vi "WPI_AnalogChannelGetSampleRate.vi"(8 "error in (no error)":errorcluster) -> (0 "error out":errorcluster, 1 "Scan List":u8[](array[numeric]), 2 "Samples Per Second":dbl)   [LabVIEW 2017]
doc: "Returns the sample rate. The effective sample rate for a channel is the sample rate divided by the number of active channels. Use the SetSampleRate VI to set the sample rate of a channel.\n\nThis software is licensed. Open the labview\\readme\\WPI Robotics Library Open Source License.txt file for more information."
uses:
  <vilib>/Rock Robotics/SystemInterfaces/System/FPGA_SystemGet.vi
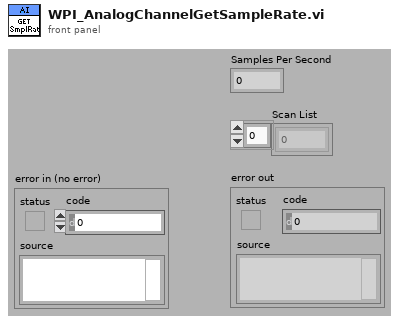
[diagram p1: front panel]
types:
  T1 = typedef "FPGA_AIDevRef.ctl" = cluster{"DevStatus":errorcluster}
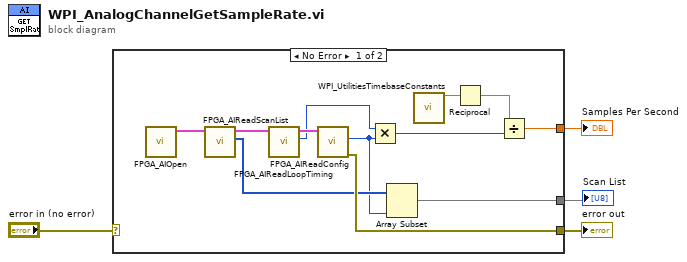
[diagram p0: block diagram]
diagram:
  n1 = case shown="No Error" "error in (no error)" {
    selector: "error in (no error)" -> [_ w17]
    tunnel: [w12 w17] -> w3
    tunnel: [w13 _] -> w2
    tunnel: [w8 _] -> w1
    frame No Error {
      n2 = call <vilib>:"FPGA_AIOpen.vi"() -> ("AI Reference out"=w11:T1)  [unwired: 3 in, 8 out]
      n3 = call <vilib>:"FPGA_AIReadScanList.vi"("AI Reference"=w11) -> ("Scan List"=w9:u8[], "AI Reference"=w10:T1)  [unwired: 1 in, 8 out]
      n4 = call <vilib>:"FPGA_AIReadLoopTiming.vi"("AI Reference"=w10) -> ("LoopTiming"=w15:u32, "AI Reference"=w16:T1)  [unwired: 1 in, 8 out]
      n5 = call <vilib>:"FPGA_AIReadConfig.vi"("AI Reference"=w16) -> ("error out"=w12:errorcluster, "Scan Size"=w7:u8)  [unwired: 1 in, 8 out]
      n6 = Multiply(x=w15, y=w7) -> (x*y=w14:u32)
      n7 = Array Subset(array=w9, length=w7) -> (w8:u8[])  [unwired: 1 in]
      n8 = call <vilib>:"WPI_UtilitiesTimebaseConstants.vi"() -> ("40 MHz FPGA clock"=w6:dbl)  [unwired: 13 in, 2 out]
      n9 = Reciprocal(x=w6) -> (1/x=w5:dbl)
      n10 = Divide(x=w5, y=w14) -> (x/y=w13:dbl)
    }
    frame Error {
    }
  }
  "Samples Per Second" <- w2
  "error out" <- w3
  "Scan List" <- w1
